vi "Number of Address Map Elements.vi"(2 "niInstr AXI4-Lite address space v1 FPGA in":refnum<class "niInstr AXI4-Lite Address Space v1 FPGA.lvclass">) -> (6 "number of elements":u8)   [LabVIEW 2015, in "niInstr AXI4-Lite Address Space v1 FPGA.lvclass"]
doc: "Returns the number of Address Map Elements contained within the address space.\n\n<B>Input Parameters</B>\n\n<B>niInstr AXI4-Lite address space v1 FPGA in</B> is the AXI4-Lite address space to use.\n\n<B>Output Parameters</B>\n\n<B>number of elements</B> is the number of Address Map Elements in the address space."
uses:
  <instrlib>/_niInstr/CLIP Adapters/v1/FPGA/AXI4-Lite/Address Space/niInstr AXI4-Lite Address Space v1 FPGA.lvclass
  <instrlib>/_niInstr/CLIP Adapters/v1/FPGA/AXI4-Lite/Address Space/niInstr AXI4-Lite Address Space v1 FPGA.lvclass/niInstr AXI4-Lite Address Space v1 FPGA.ctl
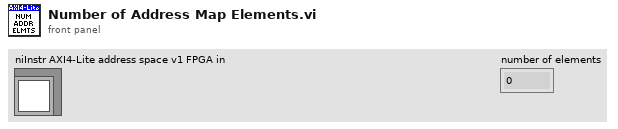
[diagram p1: front panel]
types:
  T1 = typedef "niInstr Instruction Framework v1 FPGA.lvlib/Address Map Element.ctl" = cluster{"UID":u16, "version":u16, "oldest compatible version":u16, "instance":u8, "number of children":u8, "offset":u32}
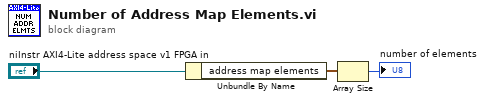
[diagram p0: block diagram]
diagram:
  n1 = Unbundle By Name("niInstr AXI4-Lite address space v1 FPGA in") -> ("address map elements"=w2:T1[])
  n2 = Array Size(array=w2) -> (size(s)=→"number of elements":i32)
